vi "UHR-Fleezers Control (host) - 12.2.vi"() -> ()   [LabVIEW 2012] (continued)
            n1564 = local write "Start Saving"(w2727) -> ()
            n1565 = Build Array("Save APD Data\nwith Trap Data", "Save Trap Pos. Data") -> (w2724:bool[])
            n1566 = Boolean Array To Number(Boolean array=w2724) -> (number=w2723:u32)
            n1567 = Build Array(w2754, w2753, w2752, w2751, w2750, w2749) -> (w2748:dbl[])
            n1568 = case shown="1, Default" w2758 {
              tunnel: w2757 -> [w2829 w2849 w2865 w2903]
              tunnel: w2728 -> [w2834 w2856 w2885 w2922]
              tunnel: w2755 -> [w2833 w2855 w2884 w2921]
              tunnel: [w2830 w2851 w2876 w2913] -> w2746
              tunnel: [w2821 "Cal sets to save" w2866 w2904] -> w2736
              tunnel: w2748 -> [w2831 w2852 w2878 w2915]
              tunnel: "Save APD Data\nwith Trap Data" -> [w2828 _ w2862 w2901]
              tunnel: [w2828 w2843 w2862 w2901] -> w2733
              tunnel: w2732 -> [w2824 w2844 w2860 w2899]
              tunnel: w2731 -> [w2823 _ _ _]
              tunnel: [w2814 w2843 w2859 w2889] -> w2720
              tunnel: "Save Trap Pos. Data" -> [w2814 _ w2859 w2889]
              tunnel: w2723 -> [w2813 _ w2858 w2888]
              frame 1, Default {
                # "timeseries"
                n1569 = case shown="True" "Profile" {
                  tunnel: [w2837 w2841] -> w2818
                  tunnel: [w2837 w2840] -> w2817
                  tunnel: [w2837 w2839] -> w2816
                  tunnel: [w2837 w2838] -> w2815
                  frame False {
                    w2837 = 0.0 ("f")
                  }
                  frame True {
                    n1570 = local read "Current Position"() -> (w2842:cluster{dbl, dbl, dbl})
                    n1571 = local read "Y change (mm)"() -> (w2838:dbl)
                    n1572 = Unbundle(w2842) -> (w2841:dbl, w2840:dbl, w2839:dbl)
                  }
                }
                n1573 = local read "Save ave N"() -> (w2836:dbl)
                n1574 = Multiply(x=w2836, y=w2829) -> (x*y=w2835:dbl)
                n1575 = To Double Precision Float(number=w2813) -> (double precision float=w2827:dbl)
                n1576 = Build Array(w2824, w2829, w2835, w2834, w2833, 0.0 ("f")) -> (w2832:dbl[])
                n1577 = Build Array(w2827, w2818, w2817, w2816, w2815) -> (w2825:dbl[])
                n1578 = Select(t=u32 4000000000, s=w2823, f="N sets to save") -> (s? t:f=w2821:u32)
                n1579 = Build Array (concatenate)(w2832, w2831, w2825) -> (w2830:dbl[])
              }
              frame 2 {
                w2846 = 0.0 ("f")
                w2843 = FALSE ("Save APD Data\nwith Trap Data")
                # "calibration"
                n1580 = Boolean To (0,1)(Boolean=w2843) -> (0, 1=w2848:i16)
                n1581 = To Double Precision Float(number=w2848) -> (double precision float=w2847:dbl)
                n1582 = Build Array(w2847, w2846, w2846, w2846, w2846) -> (w2845:dbl[])
                n1583 = Build Array(w2844, w2849, w2849, w2856, w2855, 1.0 ("t")) -> (w2853:dbl[])
                n1584 = Build Array (concatenate)(w2853, w2852, w2845) -> (w2851:dbl[])
                "Calibrating Trap..." <- TRUE ("Calibrating...")
              }
              frame 4 {
                w2863 = 0.0 ("f")
                # "scan dir (x/y = 0/1)"
                # "cycles/step"
                # "n scans (f/b)"
                # "steps"
                # "freq. range"
                # "AOD raster scan"
                n1585 = local read "Number of F/B Scans (AOD)"() -> (w2870:u16)
                n1586 = local read "Cycles/step (AOD)"() -> (w2872:u64)
                n1587 = local read "Scan Range (MHz)"() -> (w2875:dbl)
                n1588 = local read "Scan steps (AOD)"() -> (w2874:u64)
                n1589 = local read "Scan BD"() -> (w2882:bool)
                n1590 = local read "Save ave N"() -> (w2887:dbl)
                n1591 = Boolean To (0,1)(Boolean=w2882) -> (0, 1=w2881:i16)
                n1592 = To Double Precision Float(number=w2870) -> (double precision float=w2869:dbl)
                n1593 = To Double Precision Float(number=w2874) -> (double precision float=w2873:dbl)
                n1594 = To Double Precision Float(number=w2872) -> (double precision float=w2871:dbl)
                n1595 = To Double Precision Float(number=w2881) -> (double precision float=w2880:dbl)
                n1596 = Multiply(x=w2887, y=w2865) -> (x*y=w2886:dbl)
                n1597 = To Double Precision Float(number=w2858) -> (double precision float=w2864:dbl)
                n1598 = Build Array(w2864, w2863, w2863, w2863, w2863) -> (w2861:dbl[])
                n1599 = local read "N sets should be saved"() -> (w2867:dbl)
                n1600 = Build Array(w2880, w2875, w2873, w2871, w2869) -> (w2877:dbl[])
                n1601 = Build Array(w2860, w2865, w2886, w2885, w2884, 2.0 ("t")) -> (w2879:dbl[])
                n1602 = Round Toward +Infinity(x=w2867) -> (ceil(x): smallest int >= x=w2868:dbl)
                n1603 = Build Array (concatenate)(w2879, w2878, w2861, w2877) -> (w2876:dbl[])
                n1604 = To Unsigned Long Integer(number=w2868) -> (unsigned 32bit integer=w2866:u32)
              }
              frame 8 {
                w2896 = 0.0 ("f")
                # "MCL raster scan"
                n1605 = local read "Number of scans (MCL)"() -> (w2891:u64)
                n1606 = local read "Scan lines (y)"() -> (w2890:u64)
                n1607 = local read "2D or 1D Scan"() -> (w2893:bool)
                n1608 = local read "Scan Range (V)\n(of steps)"() -> (w2912:dbl)
                n1609 = local read "Fast Scan Dir"() -> (w2919:bool)
                n1610 = local read "Cycles/step (MCL)"() -> (w2909:u64)
                n1611 = local read "Scan steps (MCL)"() -> (w2911:u64)
                n1612 = Select(t=w2890, s=w2893, f=w2891) -> (s? t:f=w2892:u64)
                n1613 = Boolean To (0,1)(Boolean=w2893) -> (0, 1=w2895:i16)
                n1614 = local read "Save ave N"() -> (w2924:dbl)
                n1615 = local read "Initial X"() -> (w2898:dbl)
                n1616 = local read "Initial Y"() -> (w2897:dbl)
                n1617 = To Double Precision Float(number=w2895) -> (double precision float=w2894:dbl)
                n1618 = Boolean To (0,1)(Boolean=w2919) -> (0, 1=w2918:i16)
                n1619 = To Double Precision Float(number=w2892) -> (double precision float=w2907:dbl)
                n1620 = To Double Precision Float(number=w2911) -> (double precision float=w2910:dbl)
                n1621 = To Double Precision Float(number=w2909) -> (double precision float=w2908:dbl)
                n1622 = To Double Precision Float(number=w2918) -> (double precision float=w2917:dbl)
                n1623 = Multiply(x=w2924, y=w2903) -> (x*y=w2923:dbl)
                n1624 = To Double Precision Float(number=w2888) -> (double precision float=w2902:dbl)
                n1625 = local read "N sets should be saved (MCL)"() -> (w2905:dbl)
                n1626 = Build Array(w2902, w2894, w2896, w2896, w2896) -> (w2900:dbl[])
                n1627 = Build Array(w2917, w2912, w2910, w2908, w2907, w2898, w2897) -> (w2914:dbl[])
                n1628 = Build Array(w2899, w2903, w2923, w2922, w2921, 3.0 ("t")) -> (w2916:dbl[])
                n1629 = Round Toward +Infinity(x=w2905) -> (ceil(x): smallest int >= x=w2906:dbl)
                n1630 = Build Array (concatenate)(w2916, w2915, w2900, w2914) -> (w2913:dbl[])
                n1631 = To Unsigned Long Integer(number=w2906) -> (unsigned 32bit integer=w2904:u32)
              }
            }
            n1632 = local read "Index"() -> (w2763:dbl)
            n1633 = call "Create new save file.vi"("Insert"="", "Ext"=".dat", "Index In"=w2763) -> ("Path Out"=w2722:path, "Index Out"=w2735:dbl)
            n1634 = local write "Save file name"(w2722) -> ()
            n1635 = local write "Index"(w2735) -> ()
            n1636 = local write "Save index"(w2735) -> ()
            n1637 = Array Size(array=w2746) -> (size(s)=w2747:i32)
            n1638 = Open/Create/Replace File(file path (use dialog)=w2722, operation (0:open)=T35."create", access (0:read/write)=enum16{"read/write", "read-only", "write-only"}."write-only") -> (refnum out=w2760:refnum<file>)  [unwired: 1 in, 4 out]
            n1639 = local write "Saving..."(TRUE ("Saving...")) -> ()
            n1640 = To Double Precision Float(number=w2747) -> (double precision float=w2745:dbl)
            n1641 = String Length(string="Comment (data description)") -> (length=w2743:i32)
            n1642 = To Double Precision Float(number=w2743) -> (double precision float=w2742:dbl)
            n1643 = Deny Access(7:w2760) -> (3:w2759:refnum<file>)  [unwired: 1 in, 2 out]
            n1644 = Build Array (concatenate)(w2745, w2746, w2742) -> (w2744:dbl[])
            n1645 = case "If fluorescence data to be saved" shown="True" w2733 {
              tunnel: w2722 -> [_ w2812]
              tunnel: [refnum<k0> refnum w2792] -> w2734
              frame False {
              }
              frame True {
                w2791 = 0.0
                n1646 = local read "APD Integration Time (s)"() -> (w2797:dbl)
                n1647 = local read "N APD Samp/step"() -> (w2790:dbl)
                n1648 = Path To String(path=w2812) -> (string=w2811:string)
                n1649 = String Length(string=w2811) -> (length=w2810:i32)
                n1650 = Subtract(x=w2810, y=4) -> (x-y=w2808:i32)
                n1651 = String Subset(string=w2811, length (rest)=w2808) -> (substring=w2807:string)  [unwired: 1 out]
                n1652 = Build Array(w2797, w2790, w2791, w2791, w2791, w2791, w2791, w2791) -> (w2794:dbl[])
                n1653 = Concatenate Strings(w2807, "_fl.dat" ("string")) -> (w2805:string)
                n1654 = Array Size(array=w2794) -> (size(s)=w2796:i32)
                n1655 = String To Path(string=w2805) -> (path=w2801:path)
                n1656 = Open/Create/Replace File(file path (use dialog)=w2801, operation (0:open)=T35."create", access (0:read/write)=enum16{"read/write", "read-only", "write-only"}."write-only") -> (refnum out=w2802:refnum<file>)  [unwired: 1 in, 4 out]
                n1657 = Deny Access(7:w2802) -> (3:w2798:refnum<file>)  [unwired: 1 in, 2 out]
                n1658 = To Double Precision Float(number=w2796) -> (double precision float=w2795:dbl)
                n1659 = Build Array (concatenate)(w2795, w2794) -> (w2793:dbl[])
                n1660 = Write to Binary File(file (use dialog)=w2798, data=w2793, 5:FALSE ("prepend array or string size? (T)"), 9:T36."big-endian, network order" ("byte order (0:big-endian, network order)")) -> (refnum out=w2792:refnum<file>)  [unwired: 1 in, 3 out]
              }
            }
            n1661 = case shown="True" w2720 {
              tunnel: w2722 -> [_ w2774]
              tunnel: [refnum<k0> refnum w2773] -> w2721
              frame False {
              }
              frame True {
                w2769 = 0.0 ("element")
                n1662 = Path To String(path=w2774) -> (string=w2788:string)
                n1663 = Build Array(w2769, w2769, w2769, w2769, w2769, w2769, w2769, w2769) -> (w2770:dbl[])
                n1664 = String Length(string=w2788) -> (length=w2787:i32)
                n1665 = Subtract(x=w2787, y=4) -> (x-y=w2785:i32)
                n1666 = Array Size(array=w2770) -> (size(s)=w2772:i32)
                n1667 = String Subset(string=w2788, length (rest)=w2785) -> (substring=w2784:string)  [unwired: 1 out]
                n1668 = To Double Precision Float(number=w2772) -> (double precision float=w2771:dbl)
                n1669 = Concatenate Strings(w2784, "_pos.dat" ("string")) -> (w2782:string)
                n1670 = Build Array (concatenate)(w2771, w2770) -> (w2768:dbl[])
                n1671 = String To Path(string=w2782) -> (path=w2778:path)
                n1672 = Open/Create/Replace File(file path (use dialog)=w2778, operation (0:open)=T35."create", access (0:read/write)=enum16{"read/write", "read-only", "write-only"}."write-only") -> (refnum out=w2779:refnum<file>)  [unwired: 1 in, 4 out]
                n1673 = Deny Access(7:w2779) -> (3:w2775:refnum<file>)  [unwired: 1 in, 2 out]
                n1674 = Write to Binary File(file (use dialog)=w2775, data=w2768, 5:FALSE ("prepend array or string size? (T)"), 9:T36."big-endian, network order" ("byte order (0:big-endian, network order)")) -> (refnum out=w2773:refnum<file>)  [unwired: 1 in, 3 out]
              }
            }
            n1675 = Write to Binary File(file (use dialog)=w2759, data=w2744, 5:w2740, 9:w2738) -> (refnum out=w2741:refnum<file>)  [unwired: 1 in, 3 out]
            n1676 = Write to Binary File(file (use dialog)=w2741, data="Comment (data description)", 5:w2740, 9:w2738) -> (refnum out=w2737:refnum<file>)  [unwired: 1 in, 3 out]
          }
        }
        n1677 = feedback-in #28(w2680) -> ()
        n1678 = feedback-in #29(w2707) -> ()
        n1679 = feedback-in #30(w2679) -> ()
        n1680 = feedback-in #31(w2690) -> ()
        n1681 = feedback-in #32(w2693) -> ()
        n1682 = feedback-in #33(w2706) -> ()
        n1683 = feedback-in #34(w2696) -> ()
      }
      frame #1 {
        n1684 = local read "Saving..."() -> (w2938:bool)
        n1685 = case shown="True" w2938 {
          tunnel: w2942 -> [_ w2953]
          tunnel: w2941 -> [_ w2967]
          tunnel: w2940 -> [_ w2963]
          tunnel: w2939 -> [_ w2962]
          tunnel: w2937 -> [_ w2961]
          tunnel: w2936 -> [_ w2956]
          tunnel: w2935 -> [_ w2955]
          tunnel: w2934 -> [_ w2954]
          tunnel: w2933 -> [_ w2952]
          tunnel: w2932 -> [_ w2950]
          tunnel: w2931 -> [_ w2949]
          tunnel: w2930 -> [_ w2948]
          tunnel: w2929 -> [_ w2947]
          tunnel: w2928 -> [_ w2946]
          tunnel: w2927 -> [_ w2945]
          tunnel: w2926 -> [_ w2944]
          tunnel: w2925 -> [_ w2943]
          frame False {
          }
          frame True {
            n1686 = Multiply(x=w2953, y=w2952) -> (x*y=→"Time (s)":dbl)
            n1687 = Less Or Equal?(x=w2953, y=w2961) -> (x <= y?=w2965:bool)
            n1688 = Or(x="Stop Saving", y="Abort save 2") -> (x .or. y?=w2957:bool)
            n1689 = Not(x=w2957) -> (.not. x?=w2966:bool)
            n1690 = And(x=w2965, y=w2966) -> (x .and. y?=w2964:bool)
            n1691 = case shown="True" w2964 {
              tunnel: w2967 -> [w2974 w3049]
              tunnel: [0.0 w3052] -> w2960
              tunnel: w2953 -> [_ w3050]
              tunnel: w2961 -> [_ w3051]
              tunnel: w2963 -> [_ w3046]
              tunnel: w2962 -> [_ _]
              tunnel: w2956 -> [w2972 w3039]
              tunnel: w2955 -> [w2971 w3040]
              tunnel: w2954 -> [_ w3038]
              tunnel: w2950 -> [_ w3037]
              tunnel: w2949 -> [_ w2981]
              tunnel: w2948 -> [_ w3030]
              tunnel: w2947 -> [_ w3008]
              tunnel: w2946 -> [w2968 w2990]
              tunnel: w2945 -> [w2969 w2989]
              tunnel: w2944 -> [_ w2986]
              tunnel: w2943 -> [_ w2984]
              frame False {
                w2970 = FALSE
                n1692 = Close File(refnum=w2974) -> ()  [unwired: 1 in, 2 out]
                n1693 = case shown="True" w2971 {
                  tunnel: w2972 -> [_ w2976]
                  frame False {
                  }
                  frame True {
                    n1694 = Close File(refnum=w2976) -> ()  [unwired: 1 in, 2 out]
                  }
                }
                n1695 = case shown="True" w2968 {
                  tunnel: w2969 -> [_ w2975]
                  frame False {
                  }
                  frame True {
                    n1696 = Close File(refnum=w2975) -> ()  [unwired: 1 in, 2 out]
                  }
                }
                n1697 = local write "Raster Scanning..."(w2970) -> ()
                n1698 = local write "Calibrating Trap..."(w2970) -> ()
                n1699 = call <vilib>:"Beep.vi"() -> ()  [unwired: 3 in, 9 out]
                n1700 = local write "Stop Saving"(w2970) -> ()
                "Saving..." <- w2970
              }
              frame True {
                n1701 = local read "Calibrating Trap..."() -> (w3041:bool)
                n1702 = case "Write fl. data" shown="True" w3040 {
                  tunnel: w3039 -> [_ w3075]
                  tunnel: w3038 -> [_ w3074]
                  frame False {
                  }
                  frame True {
                    n1703 = Write to Binary File(file (use dialog)=w3075, data=w3074, 5:FALSE ("prepend array or string size? (T)"), 9:T36."big-endian, network order" ("byte order (0:big-endian, network order)")) -> ()  [unwired: 1 in, 4 out]
                  }
                }
                n1704 = Greater?(x="Save ave N", y=1.0) -> (0:w3044:bool)
                n1705 = Not(x=w3041) -> (.not. x?=w3043:bool)
                n1706 = And(x=w3043, y=w3044) -> (x .and. y?=w2987:bool)
                n1707 = case shown="True" w2987 {
                  tunnel: w2986 -> [w3055 w3066]
                  tunnel: [w3055 w3058] -> w2985
                  tunnel: "Save ave N" -> [_ w3059]
                  frame False {
                  }
                  frame True {
                    w3056 = 2 ("dimension size")
                    n1708 = Array Size(array=w3066) -> (size(s)=w3060:i32)
                    n1709 = Divide(x=w3060, y=w3056) -> (x/y=w3064:dbl)
                    n1710 = Reshape Array(w3066, w3064, w3056) -> (w3065:u64[][])
                    n1711 = Transpose 2D Array(2D array=w3065) -> (transposed array=w3063:u64[][])
                    n1712 = for {
                      tunnel: w3063 -> [w3068] mode=indexing
                      tunnel: [w3067] -> w3057 mode=indexing
                      tunnel: w3059 -> [w3069]
                      workers-P: _ -> [_]
                      n1713 = call "downsample 1D array - U64.vi"("Ave N"=w3069, "Array In"=w3068) -> ("Array Out"=w3067:u64[])  [unwired: 1 in]
                    }
                    n1714 = Transpose 2D Array(2D array=w3057) -> (transposed array=w3062:u64[][])
                    n1715 = Divide(x=w3060, y=w3059) -> (x/y=w3061:dbl)
                    n1716 = Reshape Array(w3062, w3061) -> (w3058:u64[])
                  }
                }
                n1717 = case shown="True" w2987 {
                  tunnel: w3046 -> [w3078 w3090]
                  tunnel: [w3078 w3082] -> w3042
                  tunnel: "Save ave N" -> [_ w3083]
                  tunnel: w3037 -> [_ w3081]
                  frame False {
                  }
                  frame True {
                    n1718 = Array Size(array=w3090) -> (size(s)=w3084:i32)
                    n1719 = Array Size(array=w3081) -> (size(s)=w3080:i32)
                    n1720 = Divide(x=w3084, y=w3080) -> (x/y=w3088:dbl)
                    n1721 = Reshape Array(w3090, w3088, w3080) -> (w3089:i16[][])
                    n1722 = Transpose 2D Array(2D array=w3089) -> (transposed array=w3087:i16[][])
                    n1723 = for {
                      tunnel: w3087 -> [w3093] mode=indexing
                      tunnel: [w3092] -> w3079 mode=indexing
                      tunnel: w3083 -> [w3091]
                      workers-P: _ -> [_]
                      n1724 = call "downsample 1D array - I16.vi"("Ave N"=w3091, "Array In"=w3093) -> ("Array Out"=w3092:i16[])  [unwired: 1 out]
                    }
                    n1725 = Transpose 2D Array(2D array=w3079) -> (transposed array=w3086:i16[][])
                    n1726 = Divide(x=w3084, y=w3083) -> (x/y=w3085:dbl)
                    n1727 = Reshape Array(w3086, w3085) -> (w3082:i16[])
                  }
                }
                n1728 = Index Array(array=w3008, index=1) -> (element=w3011:waveform(dbl))
                n1729 = Index Array(array=w3008, index=0) -> (element=w3013:waveform(dbl))
                n1730 = Unbundle By Name(w3011) -> ("Y"=w3015:dbl[])
                n1731 = Unbundle By Name(w3013) -> ("Y"=w3023:dbl[])
                n1732 = case "Write trap pos. data" shown="True" w2990 {
                  tunnel: w2989 -> [_ w3071]
                  tunnel: w2985 -> [_ w3070]
                  frame False {
                  }
                  frame True {
                    n1733 = Write to Binary File(file (use dialog)=w3071, data=w3070, 5:FALSE ("prepend array or string size? (T)"), 9:T36."big-endian, network order" ("byte order (0:big-endian, network order)")) -> ()  [unwired: 1 in, 4 out]
                  }
                }
                n1734 = Write to Binary File(file (use dialog)=w3049, data=w3042, 5:FALSE ("prepend array or string size? (T)"), 9:T36."big-endian, network order" ("byte order (0:big-endian, network order)")) -> ()  [unwired: 1 in, 4 out]
                n1735 = feedback #35(w3015) -> (w3017:dbl[])
                n1736 = Build Array (concatenate)(w3017, w3015) -> (w3016:dbl[])
                n1737 = Select(t=w3015, s=w2981, f=w3016) -> (s? t:f=w3001:dbl[])
                n1738 = feedback-in #35(w3001) -> ()
                n1739 = feedback #36(w3023) -> (w3036:dbl[])
                n1740 = Build Array (concatenate)(w3036, w3023) -> (w3035:dbl[])
                n1741 = Select(t=w3023, s=w2981, f=w3035) -> (s? t:f=w3010:dbl[])
                n1742 = feedback-in #36(w3010) -> ()
                n1743 = Divide(x=w3050, y=w3051) -> (x/y=w3053:dbl)
                n1744 = Multiply(x=w3053, y=100.0) -> (x*y=w3052:dbl)
                n1745 = Build Array(w3010, w3001) -> (→"Saved APD":dbl[][])
                n1746 = Array Size(array=w3010) -> (size(s)=w3028:i32)
                n1747 = Unbundle By Name(w3030) -> ("Y"=w3034:dbl[])
                n1748 = Subtract(x=w3028, y="N pts to average") -> (x-y=w3004:i32)
                n1749 = Multiply(x="N pts to average", y=u16 2) -> (x*y=w3005:u16)
                n1750 = Subtract(x=w3028, y=w3005) -> (x-y=w3003:i32)
                n1751 = feedback #37(w3034) -> (w3033:dbl[])
                n1752 = Build Array (concatenate)(w3033, w3034) -> (w3032:dbl[])
                n1753 = Select(t=w3034, s=w2981, f=w3032) -> (s? t:f=w3031:dbl[])
                "Trap Delta Graph" <- w3031
                n1754 = feedback-in #37(w3031) -> ()
                n1755 = Array Subset(array=w3010, index=w3004, length="N pts to average") -> (w3027:dbl[])
                n1756 = Array Subset(array=w3010, index=w3003, length="N pts to average") -> (w3026:dbl[])
                n1757 = Array Subset(array=w3001, index=w3004, length="N pts to average") -> (w3007:dbl[])
                n1758 = Array Subset(array=w3001, index=w3003, length="N pts to average") -> (w3006:dbl[])
                n1759 = Index Array(array=w2984, index=0) -> (element=w2982:waveform(dbl))
                n1760 = call-poly <vilib>:"Mean.vi"("X"=w3027) -> ("mean"=w3025:dbl)  [unwired: 1 out]
                n1761 = call-poly <vilib>:"Mean.vi"("X"=w3007) -> ("mean"=w3000:dbl)  [unwired: 1 out]
                n1762 = call-poly <vilib>:"Mean.vi"("X"=w3026) -> ("mean"=w3024:dbl)  [unwired: 1 out]
                n1763 = call-poly <vilib>:"Mean.vi"("X"=w3006) -> ("mean"=w2999:dbl)  [unwired: 1 out]
                n1764 = Unbundle By Name(w2982) -> ("Y"=w2979:dbl[])
                n1765 = Subtract(x=w3000, y=w2999) -> (x-y=w2991:dbl)
                "Delta Fl. 2" <- w2991
                n1766 = Subtract(x=w3025, y=w3024) -> (x-y=w3022:dbl)
                "Delta Fl. 1" <- w3022
                n1767 = Initialize Array(w3022, 1 ("dimension size")) -> (w3019:dbl[])
                n1768 = Initialize Array(w2991, 1 ("dimension size")) -> (w2996:dbl[])
                n1769 = feedback #38(w3019) -> (w3020:dbl[])
                n1770 = Build Array (concatenate)(w3020, w3019) -> (w3018:dbl[])
                n1771 = feedback #39(w2996) -> (w2997:dbl[])
                n1772 = Build Array (concatenate)(w2997, w2996) -> (w2995:dbl[])
                n1773 = feedback #40(w2979) -> (w2978:dbl[])
                n1774 = Build Array (concatenate)(w2978, w2979) -> (w2980:dbl[])
                n1775 = Select(t=w2979, s=w2981, f=w2980) -> (s? t:f=w2977:dbl[])
                "Saved trap pos" <- w2977
                n1776 = feedback-in #40(w2977) -> ()
                n1777 = Select(t=w3019, s=w2981, f=w3018) -> (s? t:f=w2994:dbl[])
                n1778 = feedback-in #38(w2994) -> ()
                n1779 = Select(t=w2996, s=w2981, f=w2995) -> (s? t:f=w2993:dbl[])
                n1780 = feedback-in #39(w2993) -> ()
                n1781 = Build Array(w2994, w2993) -> (→"Save APD Deriv":dbl[][])
              }
            }
            "Progress" <- w2960
            "Progress 2" <- w2960
          }
        }
      }
    }
    n1782 = local read "wait to reset values"() -> (w1677:bool)
    n1783 = Not(x=w1675) -> (.not. x?=w1678:bool)
    n1784 = And(x=w1678, y=w1677) -> (x .and. y?=w1679:bool)
    n1785 = case "Part of MCL raster scanning: returns to initial positions after scan done" shown="True" w1679 {
      tunnel: w1400 -> [w2500 w2507]
      tunnel: [w2500 w2506] -> w1681
      tunnel: w1399 -> [w2499 w2505]
      tunnel: [w2499 w2504] -> w1676
      frame False {
      }
      frame True {
        w2515 = 10.0 ("y")
        w2514 = 32767.0 ("y")
        # "to return scan values\nafter a synchronous \nAOM scan"
        n1786 = local read "AO2"() -> (w2508:dbl)
        n1787 = local read "AO1"() -> (w2509:dbl)
        n1788 = local write "wait to reset values"(FALSE ("wait to reset values")) -> ()
        n1789 = Multiply(x=w2509, y=w2514) -> (x*y=w2511:dbl)
        n1790 = Multiply(x=w2508, y=w2514) -> (x*y=w2513:dbl)
        n1791 = Divide(x=w2511, y=w2515) -> (x/y=w2510:dbl)
        n1792 = Divide(x=w2513, y=w2515) -> (x/y=w2512:dbl)
        n1793 = To Word Integer(number=w2510) -> (16bit integer=w2516:i16)
        n1794 = To Word Integer(number=w2512) -> (16bit integer=w2517:i16)
        n1795 = local read "Total Counts (ticks)"() -> (w2501:u32)
        n1796 = xnode "Read/Write Control"("FPGA VI Reference In"=w2507, "error in"=w2505, "AO1"=w2516, "AO2"=w2517, "MCL count"=w2501) -> ("FPGA VI Reference Out"=w2506:T19, "error out"=w2504:errorcluster)
        n1797 = local read "Scan Range (V)\n(of steps)"() -> (w2502:dbl)
        n1798 = property on="Scan Range (V)\n(of steps)" class="DigNum (strict)"("Val(Sgnl)"=w2502) -> ()  [unwired: 2 in, 2 out]
      }
    }
    n1799 = node-c288() -> ()  [unwired: 2 out]
  }
  n1800 = timed-loop "Control parameters (event loop)" {
    tunnel: w52 -> [w3102]
    shift-right: [w3101] -> _
    shift-left: errorcluster {"status"=FALSE, "code"=0, "source"=""} ("error out") -> [w3100]
    tunnel: [w3099] -> _
    timing: w137 -> [_]
    timing-out: [_] -> w136
    tunnel: w109 -> [w3098]
    tunnel: w56 -> [w3097]
    tunnel: w55 -> [w3096]
    tunnel: w54 -> [w3095]
    tunnel: w53 -> [w3094]
    stop <- w3099 stop-if-true
    n1801 = node-c288() -> ()  [unwired: 2 out]
    n1802 = event shown="[21] \"Laser interlacing mode\", \"Green Laser ON/Interlacing\", \"Red Laser ON/Interlacing\": Value Change" {
      selector: _ -> [_ _ _ _ _ _ _ _ _ _ _ _ _ _ _ _ _ _ _ _ _ _ _ _ _ _ _ _ _ _ _ _ _ _ _ _ _ _ _ _ _ _ _ _ _ _ _ _ _ _ _ _ _ _ _ _ _ _ _ _ _ _ _ _ _ _ _ _ _ _ _ _ _ _ _ _]
      dyn-events: _ -> [_ _ _ _ _ _ _ _ _ _ _ _ _ _ _ _ _ _ _ _ _ _ _ _ _ _ _ _ _ _ _ _ _ _ _ _ _ _ _ _ _ _ _ _ _ _ _ _ _ _ _ _ _ _ _ _ _ _ _ _ _ _ _ _ _ _ _ _ _ _ _ _ _ _ _ _]
      timeout: _ -> [_ _ _ _ _ _ _ _ _ _ _ _ _ _ _ _ _ _ _ _ _ _ _ _ _ _ _ _ _ _ _ _ _ _ _ _ _ _ _ _ _ _ _ _ _ _ _ _ _ _ _ _ _ _ _ _ _ _ _ _ _ _ _ _ _ _ _ _ _ _ _ _ _ _ _ _]
      tunnel: w3102 -> [w3143 _ _ _ w3181 _ w3203 _ _ _ _ w3269 _ _ w3312 w3318 w3325 w3330 w3366 w3387 w3408 w3418 _ _ w3438 w3442 w3453 w3464 w3475 w3516 w3543 w3637 w3642 w3680 _ w3715 w3719 w3730 w3734 w3738 _ w3746 _ _ _ _ _ _ _ _ _ _ _ _ _ _ _ _ _ w4124 _ w4141 _ w4148 w4166 _ w4173 w4181 w4196 w4212 w4218 _ w4227 _ w4246 _]
      tunnel: [w3142 _ _ _ w3171 _ w3202 _ _ w3234 _ w3248 _ _ w3311 w3314 w3324 w3327 w3365 w3385 w3406 w3417 _ _ w3436 _ w3447 w3458 w3469 w3510 w3541 w3635 w3640 w3678 _ w3713 w3717 w3720 w3732 w3736 _ w3744 _ _ _ _ _ _ _ _ _ _ _ _ _ _ _ _ _ w4122 _ _ _ _ w4163 _ _ _ _ _ _ _ _ _ _ _] -> w3101
      tunnel: w3100 -> [w3141 _ _ _ w3180 _ w3201 _ _ w3234 _ w3268 _ _ w3310 w3313 w3323 w3326 w3364 w3386 w3407 w3416 _ _ w3437 w3441 w3452 w3463 w3474 w3515 w3542 w3636 w3641 w3679 _ w3714 w3718 w3729 w3733 w3737 _ w3745 _ _ _ _ _ _ _ _ _ _ _ _ _ _ _ _ _ w4123 _ w4140 _ w4147 w4165 _ w4172 w4180 w4195 w4211 w4217 _ w4226 _ w4245 _]
      tunnel: [_ _ _ _ _ _ _ _ _ w3233 _ _ _ _ _ _ _ _ _ _ _ _ _ _ _ _ _ _ _ _ _ _ _ _ _ _ _ _ _ _ _ _ _ _ _ _ _ _ _ _ _ _ _ _ _ _ _ _ _ _ _ _ _ _ _ _ _ _ _ _ _ _ _ _ _ _] -> w3099
      tunnel: [_ _ _ _ _ _ _ "Round T1 X" _ _ _ _ _ _ _ _ _ _ _ _ _ _ _ _ _ _ _ _ _ _ _ _ _ _ _ _ _ _ _ _ _ _ _ _ _ _ _ _ _ _ _ _ _ _ _ _ _ _ _ _ _ _ _ _ _ _ _ _ _ _ _ _ _ _ _ _] -> _
      tunnel: [_ _ _ "Adjust Scale\nto Mean" _ _ _ _ _ _ _ _ _ _ _ _ _ _ _ _ _ _ _ _ "Test ttrig" _ _ _ _ _ _ _ _ _ _ _ _ _ _ _ _ _ _ _ _ _ _ _ _ "Flush Sample" "Flush Pump 3" "Flush Pump 1" "Clear Volume" _ _ _ _ _ _ _ _ _ _ _ _ _ _ _ _ _ _ _ _ _ _ _] -> _
      tunnel: [_ _ _ _ _ _ _ _ "Round T2 X" _ "Delayed Interlace Start" _ _ _ _ _ _ _ _ _ _ _ _ _ _ _ _ _ _ _ _ _ _ _ _ _ _ _ _ _ _ _ _ _ _ _ _ _ _ _ _ _ _ _ _ _ _ _ _ _ _ _ _ _ _ _ _ _ _ _ _ _ _ _ _ _] -> _
      tunnel: w3098 -> [_ _ _ _ _ _ _ _ _ _ _ _ _ _ _ _ _ _ _ _ _ _ _ _ _ _ _ _ _ _ _ _ _ _ _ _ _ _ _ _ _ _ _ _ _ w3903 w3910 w3917 w3922 w3931 _ _ w4037 _ _ _ _ _ _ _ _ _ _ _ _ _ _ _ _ _ _ _ _ _ _ _]
      tunnel: w3097 -> [_ _ _ _ _ _ _ _ _ _ _ _ _ _ _ _ _ _ _ _ _ _ _ _ _ _ _ _ _ _ _ _ _ _ _ _ _ _ _ _ _ _ _ w3820 _ _ _ _ _ _ w3975 _ _ w4043 _ w4052 _ w4066 _ _ _ _ _ _ _ _ _ _ _ _ _ _ _ _ _ _]
      tunnel: w3096 -> [_ _ _ _ _ _ _ _ _ _ _ _ _ _ _ _ _ _ _ _ _ _ _ _ _ _ _ _ _ _ _ _ _ _ _ _ _ _ _ _ _ _ _ _ _ _ _ _ _ _ _ _ _ _ _ _ _ _ _ _ _ _ _ _ _ _ _ _ _ _ _ _ _ _ _ _]
      tunnel: w3095 -> [_ _ _ _ _ _ _ _ _ _ _ _ _ _ _ _ _ _ _ _ _ _ _ _ _ _ _ _ _ _ _ _ _ _ _ _ _ _ _ _ _ _ w3757 _ _ _ _ _ _ _ _ w4005 _ _ w4048 _ w4059 _ w4091 _ _ _ _ _ _ _ _ _ _ _ _ _ _ _ _ _]
      tunnel: w3094 -> [_ _ _ _ _ _ _ _ _ _ _ _ _ _ _ _ _ _ _ _ _ _ _ _ _ _ _ _ _ _ _ _ _ _ _ _ _ _ _ _ _ _ _ _ _ _ _ _ _ _ _ _ _ _ _ _ _ _ _ _ _ _ _ _ _ _ _ _ _ _ _ _ _ _ _ _]
      event "AI Count (ticks)", "Sets to FIFO (Traps)", "Save ave N", "FPGA Ave.", "# Samples/channel", "N sets to save": Value Change {
        # "So that if 'Save ave N' is updated, the AOD scanning code updates too."
        n1803 = event-data() -> ()  [unwired: 6 out]
        n1804 = local read "AI Count (ticks)"() -> (w3124:u32)
        n1805 = Unbundle By Name("Sets to FIFO (Traps)") -> ("Set 1"=w3107:bool, "Set 2"=w3106:bool, "Set 3"=w3105:bool)
        n1806 = Boolean To (0,1)(Boolean="Sets to FIFO (Traps)") -> (0, 1=w3133:cluster{"Set 1":i16, "Set 2":i16, "Set 3":i16})
        n1807 = xnode "Read/Write Control"("FPGA VI Reference In"=w3143, "error in"=w3141, "ai count"=w3124, "Set 1"=w3107, "Set 2"=w3106, "Set 3"=w3105, "N of AI1 Int Acq Sets"="N Acq Sets (Traps + Fl.)") -> ("error out"=w3142:errorcluster)  [unwired: 1 out]
        n1808 = Cluster To Array(cluster=w3133) -> (array=w3132:i16[])
        n1809 = To Unsigned Long Integer(number=w3132) -> (unsigned 32bit integer=w3113:u32[])
        n1810 = local read "Scan steps (AOD)"() -> (w3134:u64)
        n1811 = Multiply(x=w3124, y="N Acq Sets (Traps + Fl.)") -> (x*y=w3122:u32)
        n1812 = Divide(x=40000000.0, y=w3124) -> (x/y=w3116:dbl)
        "AI rate (Hz)" <- w3116
        "Ave. Rate (Hz)" <- w3116
        n1813 = Add Array Elements(numeric array=w3113) -> (sum=w3125:u32)
        "Trap Sets" <- w3125
        n1814 = Reciprocal(x=w3116) -> (1/x=→"Ave. Period (s)":dbl)
        n1815 = property on="Scan steps (AOD)" class="DigNum (strict)"("Val(Sgnl)"=w3134) -> ()  [unwired: 2 in, 2 out]
        n1816 = Divide(x=w3116, y="N Acq Sets (Traps + Fl.)") -> (x/y=w3138:dbl)
        "Data Rate (Hz)" <- w3138
        n1817 = Reciprocal(x=w3138) -> (1/x=→"Data Period (s)":dbl)
        n1818 = local read "Save ave N"() -> (w3137:dbl)
        n1819 = Divide(x=w3138, y=w3137) -> (x/y=w3136:dbl)
        "Save Data Rate (Hz)" <- w3136
        n1820 = Reciprocal(x=w3136) -> (1/x=→"Save Data Period (s)":dbl)
        n1821 = Multiply(x=w3122, y="# Samples/trap") -> (x*y=w3120:u32)
        "Counts/DMA" <- w3120
        n1822 = property on="Trap Disp. Downsample" class="DigNum (strict)"("Maximum"="# Samples/trap") -> ()  [unwired: 2 in, 2 out]
        n1823 = Multiply(x=w3125, y="# Samples/trap") -> (x*y=w3114:u32)
        "# Samples/channel" <- w3114
        n1824 = Multiply(x=w3114, y=u32 8) -> (x*y=→"Trap AI Elements/DMA read":u32)
        n1825 = local read "APD Int. Count"() -> (w3121:u32)
        n1826 = Multiply(x=w3114, y=u32 3) -> (x*y=→"Trap Pos Elements/DMA read":u32)
        n1827 = Divide(x=w3120, y=w3121) -> (x/y=w3111:dbl)
        "APD Samples/FIFO Acq." <- w3111
        n1828 = Divide(x=w3120, y=40000000.0) -> (x/y=w3118:dbl)
        "DMA Update Period (s)" <- w3118
        n1829 = Multiply(x=2.0, y=w3111) -> (x*y=→"APD Elements/DMA read":dbl)
        n1830 = property on="APD Disp. Downsample" class="DigNum (strict)"("Maximum"=w3111) -> ()  [unwired: 2 in, 2 out]
        n1831 = local read "N sets to save"() -> (w3130:u32)
        n1832 = Multiply(x=w3118, y=w3130) -> (x*y=→"Total Time (s)":dbl)
        "FPGA Averaging" <- FALSE ("FPGA Averaging")
      }
      event "Remove Offset": Value Change {
        n1833 = event-data() -> ()  [unwired: 7 out]
        n1834 = local write "Remove Offset"(FALSE ("Remove Offset")) -> ()
        n1835 = local read "Bead Mean (nm)"() -> (w3145:dbl)
        n1836 = local read "Offset (nm)"() -> (w3146:dbl)
        n1837 = Add(x=w3145, y=w3146) -> (x+y=w3144:dbl)
        n1838 = local write "Offset (nm)"(w3144) -> ()
        n1839 = disable-structure shown="Disabled" {
          frame Disabled {
            n1840 = local read "Bead Mean (nm)"() -> (w3151:dbl)
            n1841 = Add(y=w3151) -> (x=w3150:dbl, x+y=w3149:dbl)
            n1842 = Subtract(x=w3151, y=w3150) -> (x-y=w3148:dbl)
            n1843 = property on="Bead Separation" class="WFChart (strict)"("YScale.Minimum"=w3148) -> ()  [unwired: 2 in, 2 out]
            n1844 = property on="Bead Separation" class="WFChart (strict)"("YScale.Maximum"=w3149) -> ()  [unwired: 2 in, 2 out]
          }
          frame Enabled {
          }
        }
      }
      event "Detector Type": Value Change {
        n1845 = event-data() -> ()  [unwired: 7 out]
        n1846 = local read "AI labels"() -> (w3152:string[])
        n1847 = property on="High Res. Display" class="Ring (strict)"("Strings []"=w3152) -> ()  [unwired: 2 in, 2 out]
        n1848 = Build Array (concatenate)(w3152, "none") -> (w3153:string[])
        n1849 = property on="FFT 1 Choice 1" class="Ring (strict)"("Strings []"=w3153) -> ()  [unwired: 2 in, 2 out]
        n1850 = property on="FFT 1 Choice 2" class="Ring (strict)"("Strings []"=w3153) -> ()  [unwired: 2 in, 2 out]
        n1851 = property on="FFT 2 Choice 1" class="Ring (strict)"("Strings []"=w3153) -> ()  [unwired: 2 in, 2 out]
        n1852 = property on="FFT 2 Choice 2" class="Ring (strict)"("Strings []"=w3153) -> ()  [unwired: 2 in, 2 out]
        n1853 = Bundle("APD 1", "APD 2") -> (w3156:cluster{string, string})  [unwired: 1 out]
        n1854 = Cluster To Array(cluster=w3156) -> (array=w3154:string[])
        n1855 = Build Array (concatenate)(w3154, w3153) -> (w3158:string[])
        n1856 = Array Size(array=w3158) -> (size(s)=w3159:i32)
        n1857 = property on="Signals to Plot" class="LstBox (strict)"("Item Names"=w3158) -> ()  [unwired: 2 in, 2 out]
        n1858 = property on="Signals to Plot" class="LstBox (strict)"("Number of Rows"=w3159) -> ()  [unwired: 2 in, 2 out]
        n1859 = property on="All Signals" class="WFChart (strict)"("LegNumRows"=w3159) -> ()  [unwired: 2 in, 2 out]
      }
      event "Adjust Scale\nto Mean": Value Change {
        n1860 = event-data() -> ()  [unwired: 7 out]
        n1861 = local read "APD 1 Rate (Hz)"() -> (w3168:dbl)
        n1862 = Multiply(x=1000.0, y="Above (kHz)") -> (x*y=w3166:dbl)
        n1863 = Multiply(x=1000.0, y="Below (kHz)") -> (x*y=w3164:dbl)
        n1864 = Add(x=w3166, y=w3168) -> (x+y=w3161:dbl)
        n1865 = Subtract(x=w3168, y=w3164) -> (x-y=w3162:dbl)
        n1866 = property on="APD Chart" class="WFChart (strict)"("YScale.Minimum"=w3162) -> ()  [unwired: 2 in, 2 out]
        n1867 = property on="APD Chart" class="WFChart (strict)"("YScale.Maximum"=w3161) -> ()  [unwired: 2 in, 2 out]
      }
      event "Phase adj. (AI1)", "+ phase (AI1)", "- phase (AI1)": Value Change {
        n1868 = event-data() -> ()  [unwired: 7 out]
        n1869 = Negate(x="Phase adj. (AI1)") -> (-x=w3178:i16)
        n1870 = Select(t=w3178, s="- phase (AI1)", f="Phase adj. (AI1)") -> (s? t:f=w3177:i16)
        n1871 = xnode "Read/Write Control"("FPGA VI Reference In"=w3181, "error in"=w3180, "Phase count adjustment"=w3177) -> ("FPGA VI Reference Out"=w3176:T19, "error out"=w3175:errorcluster)
        n1872 = Or(x="- phase (AI1)", y="+ phase (AI1)") -> (x .or. y?=w3172:bool)
        n1873 = xnode "Read/Write Control"("FPGA VI Reference In"=w3176, "error in"=w3175, "+ phase"=w3172) -> ("error out"=w3171:errorcluster)  [unwired: 1 out]
      }
      event "Signals to Plot": Double Click {
        w3184 = u32 9868950 ("Color Box")
        n1874 = event-data() -> ("Row"=w3186:i32)  [unwired: 9 out]
        n1875 = property on="All Signals" class="WFChart (strict)"("Active Plot"=w3186) -> (error out=w3197:errorcluster)  [unwired: 2 in, 1 out]
        n1876 = property on="All Signals" class="WFChart (strict)" props=["Plot", "Visible?", "Plot", "Plot Color"](error in=w3197) -> (error out=w3196:errorcluster, "Plot.Visible?"=w3195:bool)  [unwired: 1 in, 2 out]
        n1877 = Select(t=FALSE ("Plot.Visible"), s=w3195, f=TRUE ("Plot.Visible")) -> (s? t:f=w3190:bool)
        n1878 = property on="All Signals" class="WFChart (strict)"(error in=w3196, "Plot.Visible?"=w3190) -> (error out=w3192:errorcluster)  [unwired: 1 in, 1 out]
        n1879 = property on="All Signals" class="WFChart (strict)"(error in=w3192) -> (error out=w3187:errorcluster, "Plot.Plot Color"=w3191:u32)  [unwired: 1 in, 1 out]
        n1880 = property on="Signals to Plot" class="LstBox (strict)"(error in=w3187, "Active Row"=w3186) -> (error out=w3185:errorcluster)  [unwired: 1 in, 1 out]
        n1881 = Select(t=w3191, s=w3190, f=u32 0) -> (s? t:f=w3188:u32)
        n1882 = property on="Signals to Plot" class="LstBox (strict)"(error in=w3185, "CellFontColor"=w3188, "SelColor"=w3184, "CellBG"=w3184, "CellFontSize"=u32 20 ("Active Row:Cell Font:Size"), "CellFontBold"=TRUE ("Active Row:Cell Font:Bold")) -> ()  [unwired: 1 in, 2 out]
      }
      event "BD 1 Frequency 1 (MHz)", "BD 1 Frequency 2 (MHz)", "BD 1 Frequency 3 (MHz)", "BD 2 Frequency 1 (MHz)", "BD 2 Frequency 2 (MHz)", "BD 2 Frequency 3 (MHz)", "Trap Delta (MHz)": Value Change {
        n1883 = event-data() -> ("CtlRef"=w3200:refnum<vi>)  [unwired: 6 out]
        n1884 = control-ref of="Trap Delta (MHz)"() -> (w3199:refnum<vi>)
        n1885 = Equal?(x=w3199, y=w3200) -> (x = y?=w3198:bool)
        n1886 = case shown="False" "Oscillate Set 1" {
          tunnel: w3203 -> [w3223 _]
          tunnel: [w3222 w3226] -> w3202
          tunnel: w3201 -> [w3221 w3226]
          tunnel: w3198 -> [w3206 _]
          frame False {
            n1887 = local read "BD 1 Frequency 2 (MHz)"() -> (w3210:dbl)
            n1888 = local read "BD 1 Frequency 1 (MHz)"() -> (w3208:dbl)
            n1889 = Subtract(x=w3210, y="Trap Delta (MHz)") -> (x-y=w3207:dbl)
            n1890 = Select(t=w3207, s=w3206, f=w3208) -> (s? t:f=w3205:dbl)
            n1891 = local read "Y RF Frequency Limits (MHz)"() -> (w3211:T16)
            n1892 = local read "X RF Frequency Limits (MHz)"() -> (w3212:T16)
            n1893 = local read "BD 1 Frequency 3 (MHz)"() -> (w3224:dbl)
            n1894 = local write "BD 1 Frequency 1 (MHz)"(w3205) -> ()
            n1895 = local read "BD 2 Frequency 1 (MHz)"() -> (w3215:dbl)
            n1896 = local read "BD 2 Frequency 2 (MHz)"() -> (w3214:dbl)
            n1897 = local read "BD 2 Frequency 3 (MHz)"() -> (w3225:dbl)
            n1898 = call "set RF board frequency - interlace.vi"("Board 2 Frequency Limits"=w3211, "Board 1 Frequency Limits"=w3212, "error in"=w3221, "FPGA VI Reference In"=w3223, "Board 2 Frequency 3 (MHz)"=w3225, "Board 1 Frequency 3 (MHz)"=w3224, "Board 2 Frequency 2 (MHz)"=w3214, "Board 2 Frequency 1 (MHz)"=w3215, "Board 1 Frequency 2 (MHz)"=w3210, "Board 1 Frequency 1  (MHz)"=w3205) -> ("error out"=w3222:errorcluster)  [unwired: 1 out]
            n1899 = Subtract(x=w3215, y=w3214) -> (x-y=w3219:dbl)
            n1900 = Subtract(x=w3205, y=w3210) -> (x-y=w3220:dbl)
            n1901 = Square(x=w3219) -> (x^2=w3217:dbl)
            n1902 = Square(x=w3220) -> (x^2=w3218:dbl)
            n1903 = Add(x=w3218, y=w3217) -> (x+y=w3216:dbl)
            n1904 = Square Root(x=w3216) -> (sqrt(x)=w3213:dbl)
            n1905 = local write "Trap Delta (MHz)"(w3213) -> ()
            n1906 = property on="Initial delta (MHz)" class="DigNum (strict)"("Val(Sgnl)"=w3213) -> ()  [unwired: 2 in, 2 out]
          }
          frame True {
          }
        }
      }
      event "Round T1 X": Value Change {
        n1907 = event-data() -> ()  [unwired: 7 out]
        n1908 = local read "BD 1 Frequency 1 (MHz)"() -> (w3229:dbl)
        n1909 = Round To Nearest(number=w3229) -> (nearest integer value=w3228:dbl)
        n1910 = property on="BD 1 Frequency 1 (MHz)" class="DigNum (strict)"("Val(Sgnl)"=w3228) -> ()  [unwired: 2 in, 2 out]
      }
      event "Round T2 X": Value Change {
        n1911 = event-data() -> ()  [unwired: 7 out]
        n1912 = local read "BD 1 Frequency 2 (MHz)"() -> (w3231:dbl)
        n1913 = Round To Nearest(number=w3231) -> (nearest integer value=w3230:dbl)
        n1914 = property on="BD 1 Frequency 2 (MHz)" class="DigNum (strict)"("Val(Sgnl)"=w3230) -> ()  [unwired: 2 in, 2 out]
      }
      event "Stop All": Value Change {
        n1915 = event-data() -> ()  [unwired: 7 out]
        n1916 = local read "Stop All"() -> (w3233:bool)
      }
      event "Delayed Interlace Start": Value Change {
        n1917 = event-data() -> ()  [unwired: 7 out]
        n1918 = flat-sequence {
          frame #0 {
            n1919 = Multiply(x="Delay to Interlace (s)", y=1000.0) -> (x*y=w3236:dbl)
            n1920 = Wait (ms)(milliseconds to wait=w3236) -> ()  [unwired: 1 out]
          }
          frame #1 {
            n1921 = property on="Laser interlacing mode" class="RadioBtnsControl (strict)"("Val(Sgnl)"=enum32{"Laser ON", "Laser OFF", "Interlace"}."Interlace" ("Value (Signaling)")) -> ()  [unwired: 2 in, 2 out]
          }
        }
      }
      event "BD 1 Amplitude 1 (%)", "BD 1 Amplitude 2 (%)", "BD 1 Amplitude 3 (%)", "BD 2 Amplitude 1 (%)", "BD 2 Amplitude 2 (%)", "BD 2 Amplitude 3 (%)", "Trap 1 ON", "Trap 2 ON", "Trap 3 ON", "Feedback On/Off", "All FB On/Off": Value Change {
        w3260 = i16 1 ("f")
        n1922 = event-data() -> ()  [unwired: 7 out]
        n1923 = local write "Trap 1 (ON/OFF)"("Trap 1 ON") -> ()
        n1924 = local write "Trap 2 (ON/OFF)"("Trap 2 ON") -> ()
        n1925 = Boolean To (0,1)(Boolean="Trap 3 ON") -> (0, 1=w3261:i16)
        n1926 = Boolean To (0,1)(Boolean="Trap 1 ON") -> (0, 1=w3262:i16)
        n1927 = Boolean To (0,1)(Boolean="Trap 2 ON") -> (0, 1=w3263:i16)
        n1928 = Select(t=w3263, s="Trap ON/OFF X or Y Amp?", f=w3260) -> (s? t:f=w3258:i16)
        n1929 = Select(t=w3262, s="Trap ON/OFF X or Y Amp?", f=w3260) -> (s? t:f=w3259:i16)
        n1930 = Select(t=w3261, s="Trap ON/OFF X or Y Amp?", f=w3260) -> (s? t:f=w3257:i16)
        n1931 = Select(t=w3260, s="Trap ON/OFF X or Y Amp?", f=w3263) -> (s? t:f=w3255:i16)
        n1932 = Select(t=w3260, s="Trap ON/OFF X or Y Amp?", f=w3262) -> (s? t:f=w3256:i16)
        n1933 = Select(t=w3260, s="Trap ON/OFF X or Y Amp?", f=w3261) -> (s? t:f=w3254:i16)
        n1934 = And(x="All FB On/Off", y="Feedback On/Off") -> (x .and. y?=w3252:cluster{"Set 1":bool, "Set 2":bool})
        n1935 = local read "BD 1 Amplitude 1 (%)"() -> (w3272:dbl)
        n1936 = local read "BD 1 Amplitude 2 (%)"() -> (w3271:dbl)
        n1937 = local read "BD 1 Amplitude 3 (%)"() -> (w3270:dbl)
        n1938 = Unbundle By Name(w3252) -> ("Set 1"=w3247:bool, "Set 2"=w3244:bool)
        n1939 = local read "Y RF Amplitude Limits (%)"() -> (w3240:T16)
        n1940 = local read "X RF Amplitude Limits (%)"() -> (w3241:T16)
        n1941 = local read "BD 2 Amplitude 1 (%)"() -> (w3273:dbl)
        n1942 = local read "BD 2 Amplitude 2 (%)"() -> (w3274:dbl)
        n1943 = local read "BD 2 Amplitude 3 (%)"() -> (w3275:dbl)
        n1944 = And(x="Trap 2 ON", y=w3244) -> (x .and. y?=w3242:bool)
        n1945 = And(x="Trap 1 ON", y=w3247) -> (x .and. y?=w3245:bool)
        n1946 = Multiply(x=w3259, y=w3272) -> (x*y=w3267:dbl)
        n1947 = Multiply(x=w3271, y=w3258) -> (x*y=w3265:dbl)
        n1948 = Multiply(x=w3270, y=w3257) -> (x*y=w3266:dbl)
        n1949 = Multiply(x=w3273, y=w3256) -> (x*y=w3276:dbl)
        n1950 = Multiply(x=w3274, y=w3255) -> (x*y=w3277:dbl)
        n1951 = Multiply(x=w3275, y=w3254) -> (x*y=w3278:dbl)
        n1952 = call "set RF board amplitude - interlace.vi"("Board 2 Amplitude Limits"=w3240, "Board 1 Amplitude Limits"=w3241, "error in"=w3268, "FPGA VI Reference In"=w3269, "Board 2 Amplitude 3 (%)"=w3278, "Board 1 Amplitude 3 (%)"=w3266, "Board 2 Amplitude 2 (%)"=w3277, "Board 2 Amplitude 1 (%)"=w3276, "Board 1 Amplitude 2 (%)"=w3265, "Board 1 Amplitude 1 (%)"=w3267) -> ("error out"=w3249:errorcluster, "FPGA VI Reference Out"=w3250:T19)
        n1953 = xnode "Read/Write Control"("FPGA VI Reference In"=w3250, "error in"=w3249, "FB On/Off Set 1"=w3245, "FB On/Off Set 2"=w3242) -> ("error out"=w3248:errorcluster)  [unwired: 1 out]
      }
      event "Load parameters": Value Change {
        n1954 = event-data() -> ()  [unwired: 7 out]
        n1955 = property on="Saved AOD Raster Scan Parameter Sets" class="Arr (strict)"() -> ("Index Values"=w3289:u32[])  [unwired: 2 in, 2 out]
        n1956 = Index Array(array=w3289, index=0) -> (element=w3286:u32)
        n1957 = local write "Load parameters"(FALSE ("Load parameters")) -> ()
        n1958 = Index Array(array="Saved AOD Raster Scan Parameter Sets", index=w3286) -> (element=w3285:T43)
        n1959 = Unbundle By Name(w3285) -> ("Scan Range AOD (nm) 2"=w3284:dbl, "Step Size AOD (nm) 2"=w3283:dbl, "Scan Speed AOD (nm/s) 2"=w3282:dbl, "Number of scans (AOD) 2"=w3281:u16)
        n1960 = flat-sequence {
          tunnel: w3284 -> [w3292]
          tunnel: w3283 -> [w3291]
          tunnel: w3282 -> [w3290]
          tunnel: w3281 -> [w3293]
          frame #0 {
            n1961 = local write "Scan Speed (nm/s)"(w3290) -> ()
            n1962 = local write "Scan Range (nm)"(w3292) -> ()
            n1963 = local write "Step Size (nm)"(w3291) -> ()
          }
          frame #1 {
            n1964 = property on="Number of F/B Scans (AOD)" class="DigNum (strict)"("Val(Sgnl)"=w3293) -> ()  [unwired: 2 in, 2 out]
          }
        }
      }
      event "Trap 1 (ON/OFF)", "Trap 2 (ON/OFF)": Value Change {
        n1965 = event-data() -> ()  [unwired: 7 out]
        n1966 = property on="Trap 2 ON" class="Bool (strict)"("Val(Sgnl)"="Trap 2 (ON/OFF)") -> ()  [unwired: 2 in, 2 out]
        n1967 = property on="Trap 1 ON" class="Bool (strict)"("Val(Sgnl)"="Trap 1 (ON/OFF)") -> ()  [unwired: 2 in, 2 out]
      }
      event "DIO count 1 (ticks)", "DIO count 2 (ticks)", "DIO count 3 (ticks)", "Interlace", "Number Interlace Sets", "Not-Interlacing Set": Value Change {
        n1968 = event-data() -> ()  [unwired: 7 out]
        n1969 = local read "DIO count 3 (ticks)"() -> (w3306:u32)
        n1970 = local read "DIO count 1 (ticks)"() -> (w3308:u32)
        n1971 = local read "DIO count 2 (ticks)"() -> (w3307:u32)
        n1972 = To Unsigned Byte Integer(number="Not-Interlacing Set") -> (unsigned 8bit integer=w3297:u8)
        n1973 = Add(x=w3297, y=u8 1) -> (x+y=w3301:u8)
        n1974 = xnode "Read/Write Control"("FPGA VI Reference In"=w3312, "error in"=w3310, "DIO count 1 (ticks)"=w3308, "DIO count 2 (ticks)"=w3307, "DIO count 3 (ticks)"=w3306, "Interlace ON/OFF"="Interlace", "Number Interlace Cycles"="Number Interlace Sets", "Interlace Off Parameters"=w3301) -> ("error out"=w3311:errorcluster)  [unwired: 1 out]
        n1975 = Build Array(w3308, w3307, w3306) -> (w3299:u32[])
        n1976 = Split 1D Array(array=w3299, index="Number Interlace Sets") -> (first subarray=w3309:u32[])  [unwired: 1 out]
        n1977 = Index Array(array=w3299, index=w3297) -> (element=w3298:u32)
        n1978 = Add Array Elements(numeric array=w3309) -> (sum=w3303:u32)
        n1979 = Select(t=w3303, s="Interlace", f=w3298) -> (s? t:f=→"Total Counts (ticks)":u32)
      }
      event "Reset Feedback": Value Change {
        n1980 = event-data() -> ()  [unwired: 7 out]
        n1981 = Unbundle By Name("Reset Feedback") -> ("Set 1"=w3316:bool, "Set 2"=w3315:bool)
        n1982 = xnode "Read/Write Control"("FPGA VI Reference In"=w3318, "error in"=w3313, "FB Reset Set 1"=w3316, "FB Reset Set 2"=w3315) -> ("error out"=w3314:errorcluster)  [unwired: 1 out]
      }
      event "Trap Intensity PID Gains": Value Change {
        n1983 = event-data() -> ()  [unwired: 7 out]
        n1984 = Unbundle By Name("Trap Intensity PID Gains") -> ("proportional gain (Kc)"=w3321:i16, "integral gain (Kc*Ts/Ti)"=w3320:i16, "derivative gain (Kc*Td/Ts)"=w3319:i16)
        n1985 = xnode "Read/Write Control"("FPGA VI Reference In"=w3325, "error in"=w3323, "P1"=w3321, "I1"=w3320, "D1"=w3319) -> ("error out"=w3324:errorcluster)  [unwired: 1 out]
      }
      event "AI2 to Setpoint", "Setpoints (V)": Value Change {
        n1986 = event-data() -> ()  [unwired: 7 out]
        n1987 = xnode "Read/Write Control"("FPGA VI Reference In"=w3330, "error in"=w3326) -> ("FPGA VI Reference Out"=w3329:T19, "error out"=w3328:errorcluster, "AI2 Y Sum Set 1"=w3337:i16, "AI2 Y Sum Set 2"=w3336:i16)
        n1988 = Cluster To Array(cluster="AI2 to Setpoint") -> (array=w3340:bool[])
        n1989 = local read "AI2 (V)"() -> (w3338:cluster{"Set 1":dbl, "Set 2":dbl})
        n1990 = Or Array Elements(Boolean array=w3340) -> (logical OR=w3341:bool)
        n1991 = Bundle By Name(cluster=w3338, "Set 1"=w3337, "Set 2"=w3336) -> (w3335:cluster{"Set 1":dbl, "Set 2":dbl})
        n1992 = Divide(x=w3335, y=3276.7) -> (x/y=w3334:cluster{"Set 1":dbl, "Set 2":dbl})
        "AI2 (V)" <- w3334
        n1993 = case shown="True" w3341 {
          tunnel: [w3344 w3361] -> w3333
          tunnel: "AI2 to Setpoint" -> [_ w3357]
          tunnel: "Setpoints (V)" -> [w3345 w3360]
          tunnel: w3334 -> [_ w3354]
          frame False {
            n1994 = Multiply(x=3276.7, y=w3345) -> (x*y=w3346:cluster{"Set 1":dbl, "Set 2":dbl})
            n1995 = To Word Integer(number=w3346) -> (16bit integer=w3344:cluster{"Set 1":i16, "Set 2":i16})
          }
          frame True {
            n1996 = Unbundle By Name(w3354) -> ("Set 1"=w3353:dbl, "Set 2"=w3352:dbl)
            n1997 = Unbundle By Name(w3360) -> ("Set 1"=w3359:dbl, "Set 2"=w3358:dbl)
            n1998 = Unbundle By Name(w3357) -> ("Set 1"=w3356:bool, "Set 2"=w3355:bool)
            n1999 = Select(t=w3353, s=w3356, f=w3359) -> (s? t:f=w3351:dbl)
            n2000 = Select(t=w3352, s=w3355, f=w3358) -> (s? t:f=w3350:dbl)
            n2001 = Bundle By Name(cluster=w3360, "Set 1"=w3351, "Set 2"=w3350) -> (w3348:cluster{"Set 1":dbl, "Set 2":dbl})
            n2002 = local write "Setpoints (V)"(w3348) -> ()
            n2003 = Multiply(x=3276.7, y=w3348) -> (x*y=w3349:cluster{"Set 1":dbl, "Set 2":dbl})
            n2004 = To Word Integer(number=w3349) -> (16bit integer=w3361:cluster{"Set 1":i16, "Set 2":i16})
          }
        }
        n2005 = Unbundle By Name(w3333) -> ("Set 1"=w3332:i16, "Set 2"=w3331:i16)
        n2006 = xnode "Read/Write Control"("FPGA VI Reference In"=w3329, "error in"=w3328, "FB Setpoint Set 1"=w3332, "FB Setpoint Set 2"=w3331) -> ("error out"=w3327:errorcluster)  [unwired: 1 out]
      }
      event "Invert laser interlacing": Value Change {
        n2007 = event-data() -> ()  [unwired: 7 out]
        n2008 = xnode "Read/Write Control"("FPGA VI Reference In"=w3366, "error in"=w3364, "Invert GI"="Invert laser interlacing", "Invert GI 2"="Invert laser interlacing", "Invert RI"="Invert laser interlacing", "Invert RI 2"="Invert laser interlacing") -> ("error out"=w3365:errorcluster)  [unwired: 1 out]
      }
